vi "_PC_Pub_Splitter_ConfigWindow.vi"(1 "Config Tab":refnum<vi>, 2 "SplitterRef":refnum<vi>) -> ()   [LabVIEW 2018]
panel:
  in  "Dis_Param_Tab":enum32{"DAQ", "Instrument"}(tab)
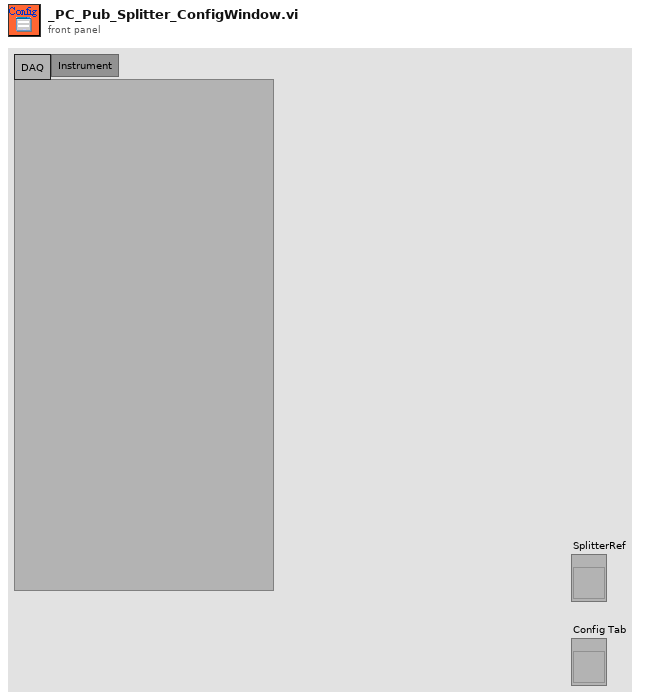
[diagram p1: front panel]
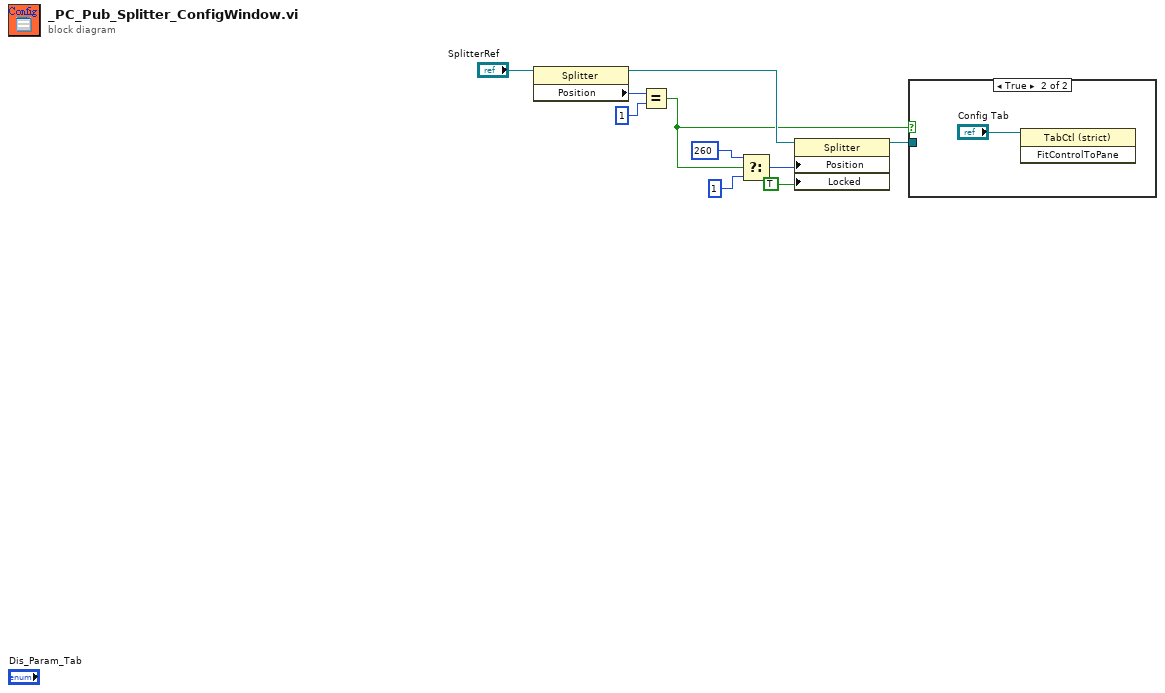
[diagram p0: block diagram]
diagram:
  n1 = property class="Splitter"(reference="SplitterRef") -> (reference out=w10:refnum<vi>, "Position"=w5:i32)  [unwired: 1 in, 1 out]
  n2 = Equal?(x=w5, y=1) -> (x = y?=w1:bool)
  n3 = Select(t=260 ("Splitter Position"), s=w1, f=1) -> (s? t:f=w4:i32)
  n4 = property class="Splitter"(reference=w10, "Position"=w4, "Locked"=TRUE ("Splitter Position Locked")) -> (reference out=w2:refnum<vi>)  [unwired: 1 in, 1 out]
  n5 = case shown="True" w1 {
    tunnel: w2 -> [_ _]
    frame False {
    }
    frame True {
      n6 = invoke class="TabCtl (strict)" method="FitControlToPane"(reference="Config Tab") -> ()  [unwired: 2 in, 3 out]
    }
  }
